vi "Trigger Home Screen.vi"() -> ()   [LabVIEW 2017]
panel:
  out "Trigger Home Screen":bool
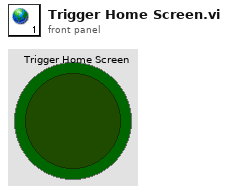
[diagram p1: front panel]
diagram:
